vi "氨氮加标回收.vi"   [LabVIEW 2016, in "质控单元.lvlib"]
types:
  T1 = enum16{"init", "采配水运行", "加标前测水样", "加标", "加标后测水样", "计算", "结束"}
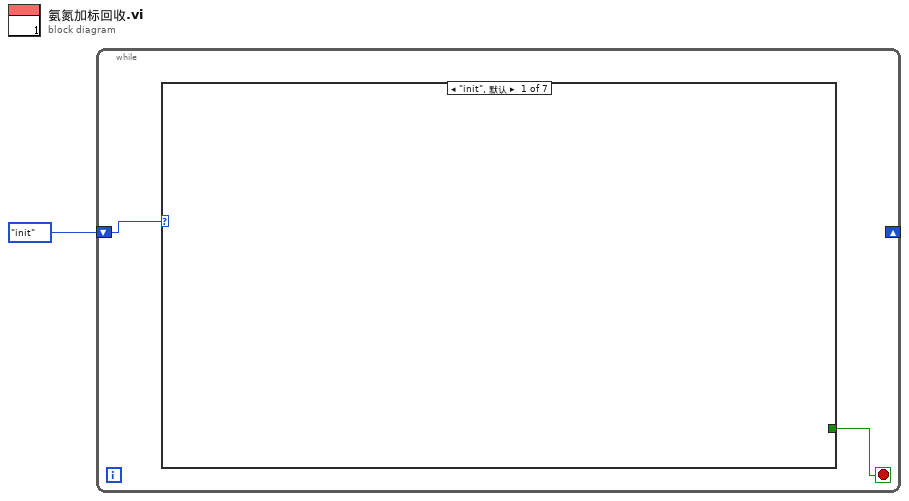
[diagram p0: block diagram]
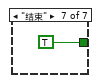
[diagram p7: hidden frame]
diagram:
  n1 = while {
    shift-right: _ -> [_]
    shift-left: T1."init" ("枚举") -> [w3]
    stop <- w2 stop-if-true
    n2 = case shown="\"init\", 默认" w3 {
      tunnel: [_ _ _ _ _ _ TRUE] -> w2
      frame "init", Default {
      }
      frame "采配水运行" {
      }
      frame "加标前测水样" {
      }
      frame "加标" {
      }
      frame "加标后测水样" {
      }
      frame "计算" {
      }
      frame "结束" {
      }
    }
  }
